vi "Calc Phase Shift.vi"(10 "Signal 2":waveform(dbl), 11 "Signal 1":waveform(dbl)) -> (0 "magnitude":dbl, 1 "Freq":dbl=0.3, 2 "Phase Shift":dbl, 3 "Time Shift":dbl)   [LabVIEW 2011]
uses:
  <vilib>/Analysis/NI_AALPro.lvlib
  <vilib>/measure/NI_MABase.lvlib
panel:
  out "signal b":waveform(dbl)(graph)
  in  "phase":dbl format="%.2p"
  out "signal a":waveform(dbl)(graph)
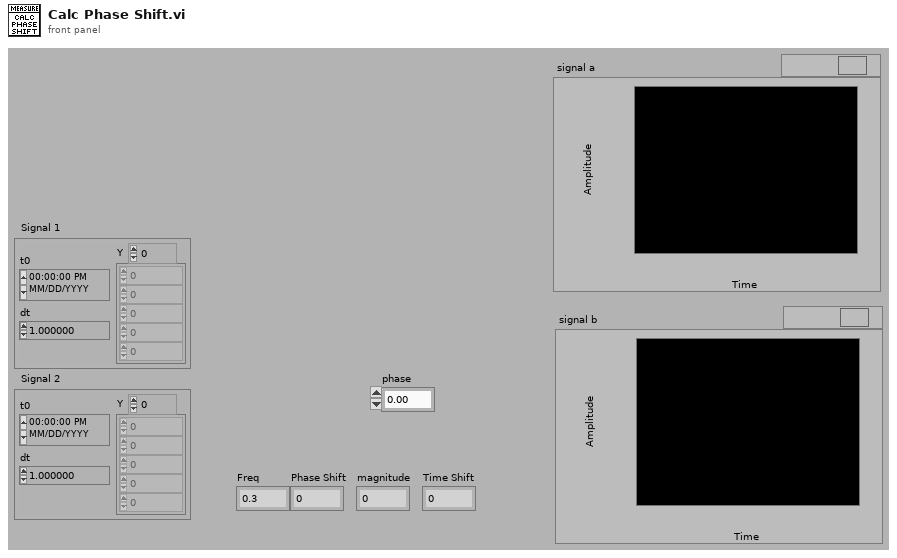
[diagram p1: front panel]
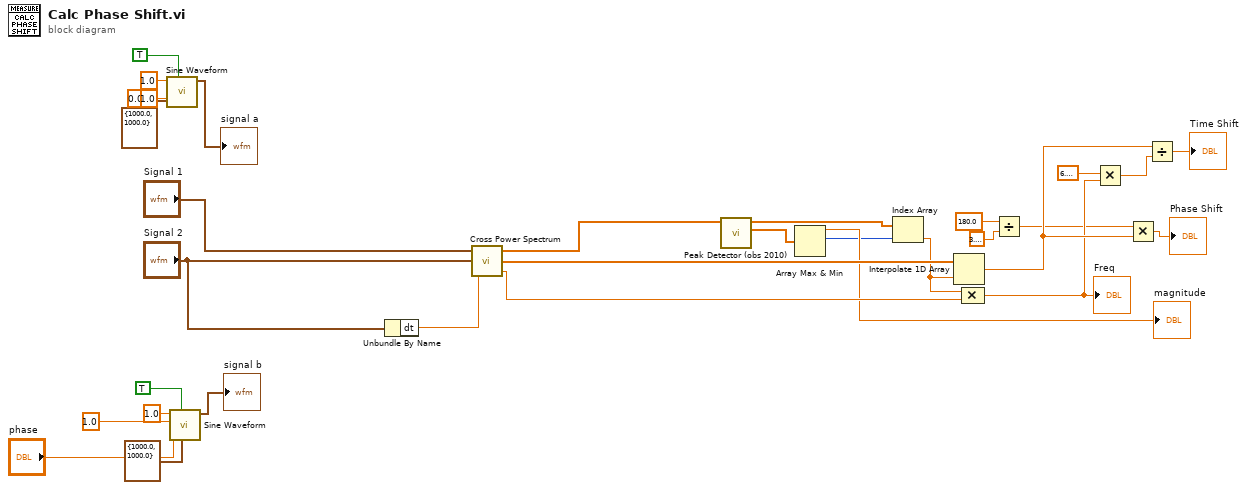
[diagram p0: block diagram]
diagram:
  n1 = call <vilib>:"Sine Waveform.vi"("sampling info"=cluster{"Fs":dbl, "#s":dbl} {"Fs"=1000.0, "#s"=1000.0}, "reset signal"=TRUE, "phase"=0.0, "amplitude"=1.0, "frequency"=1.0) -> ("signal out"=→"signal a":waveform(dbl))  [unwired: 5 in, 1 out]
  n2 = call <vilib>:"Sine Waveform.vi"("sampling info"=cluster{"Fs":dbl, "#s":dbl} {"Fs"=1000.0, "#s"=1000.0}, "reset signal"=TRUE, "phase"="phase", "amplitude"=1.0, "frequency"=1.0) -> ("signal out"=→"signal b":waveform(dbl))  [unwired: 5 in, 1 out]
  n3 = Unbundle By Name("Signal 2") -> ("dt"=w25:dbl)
  n4 = call <vilib>:"Cross Power Spectrum.vi"("dt"=w25, "Signal Y (V)"="Signal 2", "Signal X (V)"="Signal 1") -> ("df"=w29:dbl, "Cross Power XY Spectrum Phase (radians)"=w30:dbl[], "Cross Power XY Spectrum Mag (V^2rms)"=w28:dbl[])
  n5 = call <vilib>:"Peak Detector (obs 2010).vi"("X"=w28) -> ("Amplitudes"=w17:dbl[], "Locations"=w27:dbl[])  [unwired: 6 in, 3 out]
  n6 = Array Max & Min(array=w17) -> (max value=→"magnitude":dbl, max index (indices)=w16:i32)  [unwired: 2 out]
  n7 = Index Array(array=w27, index=w16) -> (element=w15:dbl)
  n8 = Interpolate 1D Array(1:w15, 2:w30) -> (0:w24:dbl)
  n9 = Compound Arithmetic op=MULTIPLY(w15, w29) -> (w22:dbl)
  "Freq" <- w22
  n10 = Divide(x=180.0, y=3.141592653589793) -> (x/y=w18:dbl)
  n11 = Multiply(x=6.283185307179586, y=w22) -> (x*y=w21:dbl)
  n12 = Multiply(x=w18, y=w24) -> (x*y=→"Phase Shift":dbl)
  n13 = Divide(x=w24, y=w21) -> (x/y=→"Time Shift":dbl)
